vi "file_name_path_conv_sub.vi"(2 "Add_No":i32, 3 "Add_Str":string, 4 "path_In":path) -> (1 "path_Out":path)   [LabVIEW 2021]
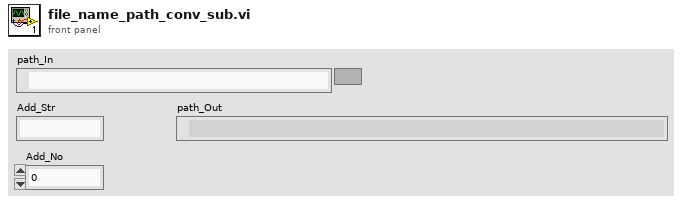
[diagram p1: front panel]
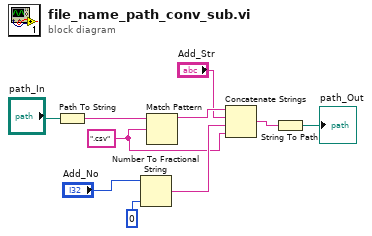
[diagram p0: block diagram]
diagram:
  w3 = ".csv" ("정규식")
  n1 = Path To String(path="path_In") -> (string=w6:string)
  n2 = Number To Fractional String(number="Add_No", precision (6)=0) -> (F-format string=w5:string)  [unwired: 2 in]
  n3 = Match Pattern(string=w6, regular expression=w3) -> (before substring=w2:string)  [unwired: 1 in, 3 out]
  n4 = Concatenate Strings(w2, "Add_Str", w5, w3) -> (w4:string)
  n5 = String To Path(string=w4) -> (path=→"path_Out":path)
